vi "Convert Set To Array.vi"   [LabVIEW 2020]
doc: "Places the code that you can use to convert a set to an array."
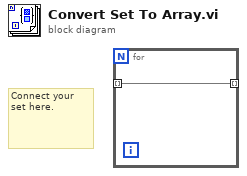
[diagram p0: block diagram]
diagram:
  # "Connect your set here."
  n1 = for {
    tunnel: [w1] -> _ mode=indexing
    tunnel: _ -> [w1] mode=indexing
  }
